vi "Begin.vi"(8 "error in":errorcluster) -> (0 "error out":errorcluster)   [LabVIEW 2020]
doc: "Called before other user functions, this VI is expected to open initial I/O refnums, load in file data, and do all program initialization. Notice that the <B>error out</B> terminal is simply used for data flow. Wiring it to other structures or subVIs ensures that this VI runs first."
uses:
  <vilib>/Rock Robotics/WPI/Joystick/WPI_JoystickDeviceEnum.ctl
  <vilib>/Rock Robotics/SystemInterfaces/spilib/spi_bus.ctl
  <vilib>/Rock Robotics/SystemInterfaces/DIO/FPGA_DIOPWMChannel.ctl
  <vilib>/Rock Robotics/WPI/RobotDrive/WPI_RobotDriveDevRef.ctl
  <vilib>/Rock Robotics/WPI/MotorControl/WPI_MotorControlDeviceRef.ctl
  <vilib>/Rock Robotics/WPI/MotorControl/WPI_MotorControlType.ctl
  <vilib>/Rock Robotics/WPI/PWM/WPI_PWMDeadband.ctl
  <vilib>/Rock Robotics/SystemInterfaces/DIO/FPGA_DIOChannel.ctl
  <vilib>/Rock Robotics/WPI/SafetyOutput/WPI_SafetyOutputConfigMenu.ctl
  <vilib>/Rock Robotics/WPI/DriverStation/WPI_DriverStationRobotMode2.ctl
  <vilib>/Rock Robotics/WPI/Gyro/WPI_GyroXRS450_SPI_Open.vi
  <vilib>/Rock Robotics/Network Tables/NT Write String Array.vi
  Robot Global Data.vi
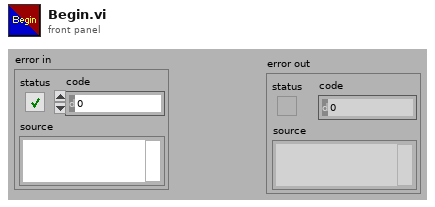
[diagram p1: front panel]
types:
  T1 = typedef "WPI_DriverStationRobotMode2.ctl" = enum16{"Autonomous Disabled", "Autonomous Enabled", "Teleop Disabled", "Teleop Enabled", "Disconnected", "Finish", "Test Disabled", "Test Enabled", "Emergency Stopped"}
  T2 = typedef "WPI_SafetyOutputConfigMenu.ctl" = enum16{"Enable", "Disable"}
  T3 = typedef "WPI_RobotDriveDevRef.ctl" = cluster{"DevStatus":errorcluster, "Motors[]":T4[], "Square Inputs":bool, "Max Output":dbl}
  T4 = typedef "WPI_MotorControlDeviceRef.ctl" = cluster{"DeviceStatus":errorcluster, "Type":T5, "PWM":cluster{"PWM Channel":T6, "DeadBand":T7}, "CAN":cluster{"Device Number":u8, "SetOutput VI Ref":variant, "GetOutput VI Ref":variant, "Enable VI Ref":variant, "Disable VI Ref":variant, "Data":variant}, "Invert":bool, "DIO PWM":cluster{"PWM \"Enable\" Channel":T6, "DIOChannel":T8, "PWM Rate":dbl}}
  T5 = typedef "WPI_MotorControlType.ctl" = enum16{"PWM", "CAN", "DIO PWM"}
  T6 = typedef "FPGA_DIOPWMChannel.ctl" = enum8{"PWM 0", "PWM 1", "PWM 2", "PWM 3", "PWM 4", "PWM 5", "PWM 6", "PWM 7", "PWM 8", "PWM 9", "PWM MXP 0", "PWM MXP 1", "PWM MXP 2", "PWM MXP 3", "PWM MXP 4", "PWM MXP 5", "PWM MXP 6", "PWM MXP 7", "PWM MXP 8", "PWM MXP 9", "Invalid"}
  T7 = typedef "WPI_PWMDeadband.ctl" = cluster{"Name":string, "maxPositivePwm":i32, "minPositivePwm":i32, "centerPwm":i32, "maxNegativePwm":i32, "minNegativePwm":i32, "angularRange":u16}
  T8 = typedef "FPGA_DIOChannel.ctl" = enum8{"DIO 0", "DIO 1", "DIO 2", "DIO 3", "DIO 4", "DIO 5", "DIO 6", "DIO 7", "DIO 8", "DIO 9", "DIO MXP 0", "DIO MXP 1", "DIO MXP 2", "DIO MXP 3", "DIO MXP 4", "DIO MXP 5", "DIO MXP 6", "DIO MXP 7", "DIO MXP 8", "DIO MXP 9", "DIO MXP 10", "DIO MXP 11", "DIO MXP 12", "DIO MXP 13", "DIO MXP 14", "DIO MXP 15", "SPI Port CS1", "SPI Port CS2", "SPI Port CS3", "SPI Port MISO", "SPI Port MOSI", "Invalid"}
  T9 = typedef "spi_bus.ctl" = enum16{"SPI On-Board, CS0", "SPI On-Board, CS1", "SPI On-Board, CS2", "SPI On-Board, CS3", "SPI MXP", "Invalid"}
  T10 = typedef "WPI_JoystickDeviceEnum.ctl" = enum16{"USB 0", "USB 1", "USB 2", "USB 3", "USB 4", "USB 5"}
  T11 = typedef "WPI_GyroDevRef.ctl" = cluster{"DevStatus":errorcluster, "Analog Channel":T12, "Gain (VoltsPerDegree/Second)":dbl, "Gyro Type":enum16{"Analog", "XRS450"}, "Handle":i32, "SPI Bus":T9, "Device Found":bool, "Sample Rate":dbl, "Calibrate On Open":bool, "Offset":dbl}
  T12 = typedef "FPGA_AIChannel.ctl" = enum8{"AI 0", "AI 1", "AI 2", "AI 3", "AI MXP 0", "AI MXP 1", "AI MXP 2", "AI MXP 3", "Invalid"}
  T13 = typedef "WPI_ServoDeviceRef.ctl" = cluster{"DeviceStatus":errorcluster, "PWM Channel":T6, "DeadBand":T7}
  T14 = typedef "WPI_JoystickDevRef.ctl" = cluster{"Device":T10}
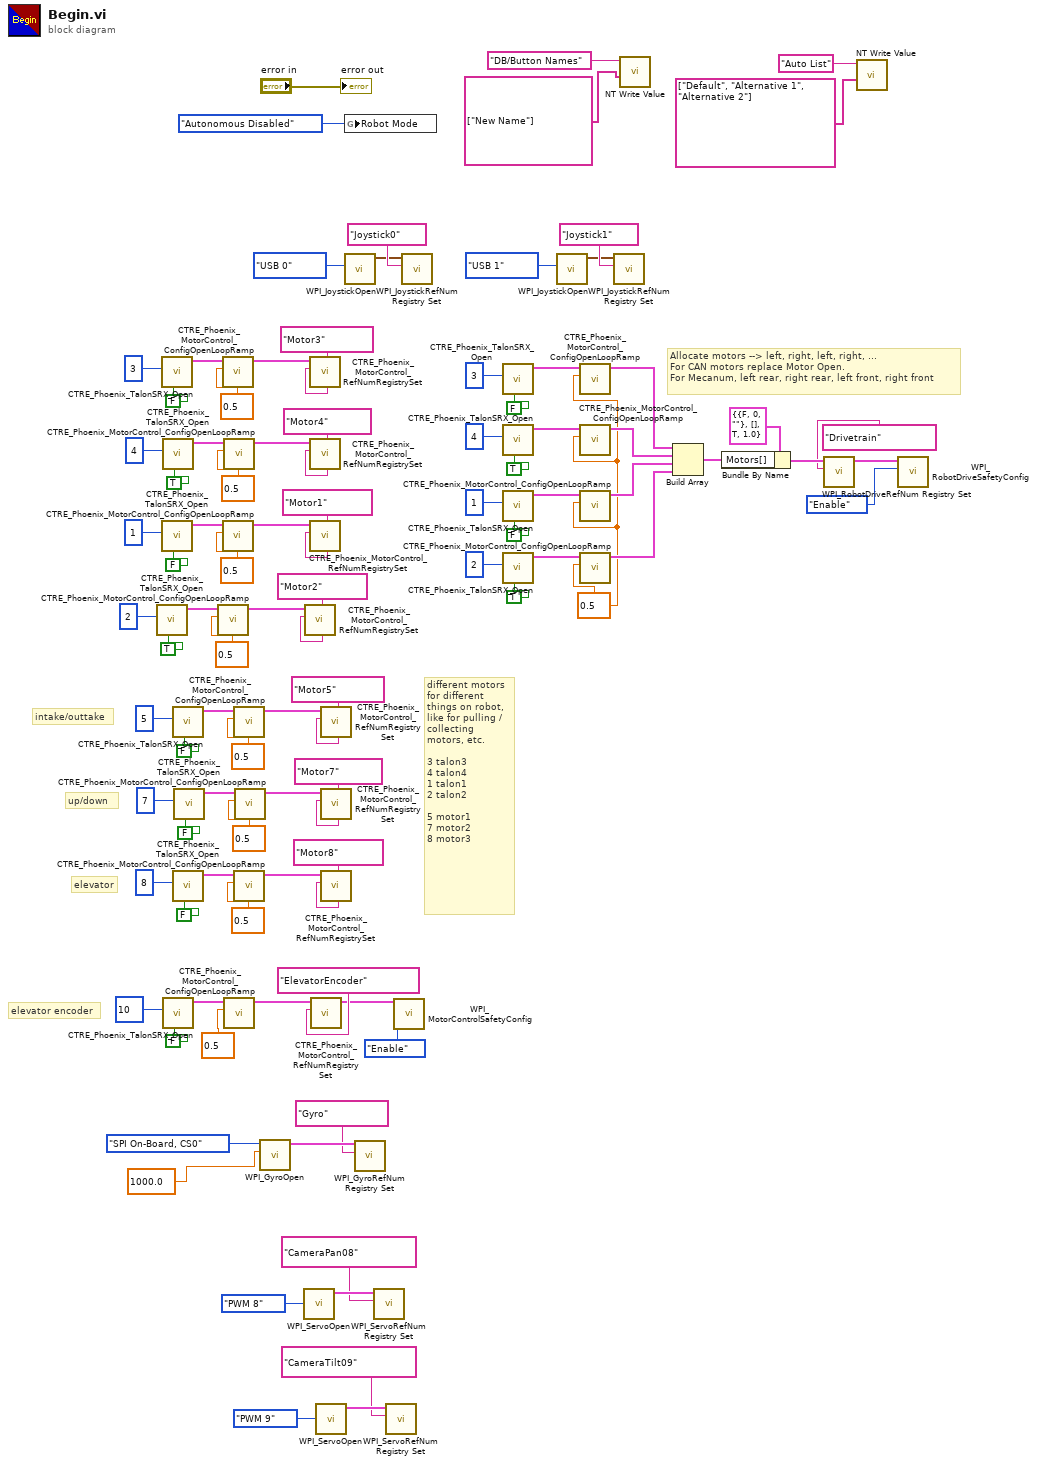
[diagram p0: block diagram]
diagram:
  w23 = 0.5 ("secondsFromNeutralToFull")
  # "elevator encoder"
  # "Allocate motors --> left, right, left, right, ... \nFor CAN motors replace Motor Open.\nFor Mecanum, left rear, right rear, left front, right front"
  # "elevator"
  # "up/down"
  # "intake/outtake"
  # "different motors for different things on robot, like for pulling / collecting motors, etc.\n\n3 talon3\n4 talon4\n1 talon1\n2 talon2\n\n5 motor1\n7 motor2\n8 motor3"
  n1 = call <vilib>:"CTRE_Phoenix_TalonSRX_Open.vi"("Invert"=TRUE, "Device Number"=u8 2) -> ("PhoenixMotorControlDevRef"=w42:T4)  [unwired: 8 in, 1 out]
  n2 = call <vilib>:"CTRE_Phoenix_TalonSRX_Open.vi"("Invert"=FALSE, "Device Number"=u8 3) -> ("PhoenixMotorControlDevRef"=w60:T4)  [unwired: 8 in, 1 out]
  n3 = call <vilib>:"CTRE_Phoenix_TalonSRX_Open.vi"("Invert"=FALSE, "Device Number"=u8 1) -> ("PhoenixMotorControlDevRef"=w56:T4)  [unwired: 8 in, 1 out]
  n4 = call <vilib>:"CTRE_Phoenix_TalonSRX_Open.vi"("Invert"=TRUE, "Device Number"=u8 4) -> ("PhoenixMotorControlDevRef"=w58:T4)  [unwired: 8 in, 1 out]
  n5 = call <vilib>:"CTRE_Phoenix_TalonSRX_Open.vi"("Invert"=FALSE, "Device Number"=u8 10) -> ("PhoenixMotorControlDevRef"=w9:T4)  [unwired: 8 in, 1 out]
  n6 = call <vilib>:"CTRE_Phoenix_TalonSRX_Open.vi"("Invert"=FALSE, "Device Number"=u8 5) -> ("PhoenixMotorControlDevRef"=w88:T4)  [unwired: 8 in, 1 out]
  n7 = call <vilib>:"CTRE_Phoenix_TalonSRX_Open.vi"("Invert"=FALSE, "Device Number"=u8 8) -> ("PhoenixMotorControlDevRef"=w84:T4)  [unwired: 8 in, 1 out]
  n8 = call <vilib>:"CTRE_Phoenix_TalonSRX_Open.vi"("Invert"=FALSE, "Device Number"=u8 7) -> ("PhoenixMotorControlDevRef"=w86:T4)  [unwired: 8 in, 1 out]
  n9 = call <vilib>:"CTRE_Phoenix_MotorControl_ConfigOpenLoopRamp.vi"("secondsFromNeutralToFull"=0.5, "PhoenixMotorControlDevRef"=w42) -> ("PhoenixMotorControlDevRef"=w40:T4)  [unwired: 8 in, 1 out]
  n10 = call <vilib>:"CTRE_Phoenix_MotorControl_ConfigOpenLoopRamp.vi"("secondsFromNeutralToFull"=0.5, "PhoenixMotorControlDevRef"=w60) -> ("PhoenixMotorControlDevRef"=w54:T4)  [unwired: 8 in, 1 out]
  n11 = call <vilib>:"CTRE_Phoenix_MotorControl_ConfigOpenLoopRamp.vi"("secondsFromNeutralToFull"=0.5, "PhoenixMotorControlDevRef"=w56) -> ("PhoenixMotorControlDevRef"=w52:T4)  [unwired: 8 in, 1 out]
  n12 = call <vilib>:"CTRE_Phoenix_MotorControl_ConfigOpenLoopRamp.vi"("secondsFromNeutralToFull"=0.5, "PhoenixMotorControlDevRef"=w58) -> ("PhoenixMotorControlDevRef"=w53:T4)  [unwired: 8 in, 1 out]
  n13 = call <vilib>:"CTRE_Phoenix_MotorControl_ConfigOpenLoopRamp.vi"("secondsFromNeutralToFull"=0.5, "PhoenixMotorControlDevRef"=w9) -> ("PhoenixMotorControlDevRef"=w7:T4)  [unwired: 8 in, 1 out]
  n14 = call <vilib>:"CTRE_Phoenix_MotorControl_ConfigOpenLoopRamp.vi"("secondsFromNeutralToFull"=0.5, "PhoenixMotorControlDevRef"=w88) -> ("PhoenixMotorControlDevRef"=w82:T4)  [unwired: 8 in, 1 out]
  n15 = call <vilib>:"CTRE_Phoenix_MotorControl_ConfigOpenLoopRamp.vi"("secondsFromNeutralToFull"=0.5, "PhoenixMotorControlDevRef"=w84) -> ("PhoenixMotorControlDevRef"=w80:T4)  [unwired: 8 in, 1 out]
  n16 = call <vilib>:"CTRE_Phoenix_MotorControl_ConfigOpenLoopRamp.vi"("secondsFromNeutralToFull"=0.5, "PhoenixMotorControlDevRef"=w86) -> ("PhoenixMotorControlDevRef"=w81:T4)  [unwired: 8 in, 1 out]
  n17 = call-poly <vilib>:"WPI_GyroOpen.vi"("Sample Rate (Hz)"=1000.0 ("secondsFromNeutralToFull"), "SPI Bus"=spi_bus."SPI On-Board, CS0") -> ("GyroDevRef"=w70:T11)  [unwired: 7 in, 2 out]
  n18 = call <vilib>:"WPI_ServoOpen.vi"("PWM Channel"=FPGA_DIOPWMChannel."PWM 8" ("PWMChannel")) -> ("ServoDeviceRef"=w66:T13)  [unwired: 9 in, 1 out]
  n19 = call <vilib>:"CTRE_Phoenix_MotorControl_RefNumRegistrySet.vi"("refnum name"="Motor2", "PhoenixMotorControlDevRef"=w40) -> ()  [unwired: 8 in, 2 out]
  n20 = call <vilib>:"CTRE_Phoenix_MotorControl_RefNumRegistrySet.vi"("refnum name"="Motor3", "PhoenixMotorControlDevRef"=w54) -> ()  [unwired: 8 in, 2 out]
  n21 = call <vilib>:"CTRE_Phoenix_MotorControl_RefNumRegistrySet.vi"("refnum name"="Motor4", "PhoenixMotorControlDevRef"=w53) -> ()  [unwired: 8 in, 2 out]
  n22 = call <vilib>:"CTRE_Phoenix_MotorControl_RefNumRegistrySet.vi"("refnum name"="Motor1", "PhoenixMotorControlDevRef"=w52) -> ()  [unwired: 8 in, 2 out]
  n23 = call <vilib>:"CTRE_Phoenix_MotorControl_RefNumRegistrySet.vi"("refnum name"="ElevatorEncoder", "PhoenixMotorControlDevRef"=w7) -> ("PhoenixMotorControlDevRef"=w3:T4)  [unwired: 8 in, 1 out]
  n24 = call <vilib>:"WPI_ServoOpen.vi"("PWM Channel"=FPGA_DIOPWMChannel."PWM 9" ("PWMChannel")) -> ("ServoDeviceRef"=w63:T13)  [unwired: 9 in, 1 out]
  n25 = call <vilib>:"CTRE_Phoenix_MotorControl_RefNumRegistrySet.vi"("refnum name"="Motor5", "PhoenixMotorControlDevRef"=w82) -> ()  [unwired: 8 in, 2 out]
  n26 = call <vilib>:"CTRE_Phoenix_MotorControl_RefNumRegistrySet.vi"("refnum name"="Motor7", "PhoenixMotorControlDevRef"=w81) -> ()  [unwired: 8 in, 2 out]
  n27 = call <vilib>:"CTRE_Phoenix_MotorControl_RefNumRegistrySet.vi"("refnum name"="Motor8", "PhoenixMotorControlDevRef"=w80) -> ()  [unwired: 8 in, 2 out]
  n28 = global write "Robot Global Data.vi" "Robot Mode"(WPI_DriverStationRobotMode2."Autonomous Disabled" ("Robot Mode")) -> ()
  n29 = call <vilib>:"WPI_JoystickOpen.vi"("JoystickDevice"=WPI_JoystickDeviceEnum."USB 0") -> ("JoystickDevRef"=w94:T14)  [unwired: 10 in]
  n30 = call <vilib>:"WPI_GyroRefNum Registry Set.vi"("refnum name"="Gyro", "GyroDevRef"=w70) -> ()  [unwired: 8 in, 2 out]
  n31 = call <vilib>:"WPI_ServoRefNum Registry Set.vi"("refnum name"="CameraPan08", "ServoDeviceRef"=w66) -> ()  [unwired: 8 in, 2 out]
  n32 = call <vilib>:"WPI_ServoRefNum Registry Set.vi"("refnum name"="CameraTilt09", "ServoDeviceRef"=w63) -> ()  [unwired: 8 in, 2 out]
  n33 = call <vilib>:"WPI_MotorControlSafetyConfig.vi"("mode"=WPI_SafetyOutputConfigMenu."Enable", "MotorControlDevRef"=w3) -> ()  [unwired: 8 in, 2 out]
  n34 = call <vilib>:"WPI_JoystickRefNum Registry Set.vi"("refnum name"="Joystick0", "JoystickDevRef"=w94) -> ()  [unwired: 8 in, 2 out]
  n35 = call <vilib>:"CTRE_Phoenix_TalonSRX_Open.vi"("Invert"=FALSE, "Device Number"=u8 3) -> ("PhoenixMotorControlDevRef"=w31:T4)  [unwired: 8 in, 1 out]
  n36 = call <vilib>:"CTRE_Phoenix_TalonSRX_Open.vi"("Invert"=TRUE, "Device Number"=u8 4) -> ("PhoenixMotorControlDevRef"=w30:T4)  [unwired: 8 in, 1 out]
  n37 = call <vilib>:"CTRE_Phoenix_TalonSRX_Open.vi"("Invert"=FALSE, "Device Number"=u8 1) -> ("PhoenixMotorControlDevRef"=w29:T4)  [unwired: 8 in, 1 out]
  n38 = call <vilib>:"CTRE_Phoenix_TalonSRX_Open.vi"("Invert"=TRUE, "Device Number"=u8 2) -> ("PhoenixMotorControlDevRef"=w28:T4)  [unwired: 8 in, 1 out]
  n39 = call <vilib>:"WPI_JoystickOpen.vi"("JoystickDevice"=WPI_JoystickDeviceEnum."USB 1") -> ("JoystickDevRef"=w90:T14)  [unwired: 10 in]
  n40 = call <vilib>:"CTRE_Phoenix_MotorControl_ConfigOpenLoopRamp.vi"("secondsFromNeutralToFull"=w23, "PhoenixMotorControlDevRef"=w31) -> ("PhoenixMotorControlDevRef"=w26:T4)  [unwired: 8 in, 1 out]
  n41 = call <vilib>:"CTRE_Phoenix_MotorControl_ConfigOpenLoopRamp.vi"("secondsFromNeutralToFull"=w23, "PhoenixMotorControlDevRef"=w30) -> ("PhoenixMotorControlDevRef"=w25:T4)  [unwired: 8 in, 1 out]
  n42 = call <vilib>:"CTRE_Phoenix_MotorControl_ConfigOpenLoopRamp.vi"("secondsFromNeutralToFull"=w23, "PhoenixMotorControlDevRef"=w29) -> ("PhoenixMotorControlDevRef"=w24:T4)  [unwired: 8 in, 1 out]
  n43 = call <vilib>:"CTRE_Phoenix_MotorControl_ConfigOpenLoopRamp.vi"("secondsFromNeutralToFull"=w23, "PhoenixMotorControlDevRef"=w28) -> ("PhoenixMotorControlDevRef"=w27:T4)  [unwired: 8 in, 1 out]
  n44 = call <vilib>:"WPI_JoystickRefNum Registry Set.vi"("refnum name"="Joystick1", "JoystickDevRef"=w90) -> ()  [unwired: 8 in, 2 out]
  n45 = call-poly <vilib>:"NT Write Value.vi"("String Array"=string[] ["New Name"], "Name"="DB/Button Names") -> ()  [unwired: 9 in, 1 out]
  n46 = Build Array(w26, w25, w24, w27) -> (w22:T4[])
  n47 = Bundle By Name(cluster=T3 {"DevStatus"={"status"=FALSE, "code"=0, "source"=""}, "Motors[]"=[], "Square Inputs"=TRUE, "Max Output"=1.0} ("RobotDriveDevRef"), "Motors[]"=w22) -> (w34:T3)
  n48 = call <vilib>:"WPI_RobotDriveRefNum Registry Set.vi"("refnum name"="Drivetrain", "RobotDriveDevRef"=w34) -> ("RobotDriveDevRef"=w33:T3)  [unwired: 8 in, 1 out]
  n49 = call-poly <vilib>:"NT Write Value.vi"("String Array"=string[] ["Default", "Alternative 1", "Alternative 2"], "Name"="Auto List") -> ()  [unwired: 9 in, 1 out]
  n50 = call <vilib>:"WPI_RobotDriveSafetyConfig.vi"("mode"=WPI_SafetyOutputConfigMenu."Enable", "RobotDriveDevRef"=w33) -> ()  [unwired: 2 in, 8 out]
  "error out" <- "error in"
